vi "Obtain frame number and location-single bin file.vi"(8 "error in (no error)":errorcluster, 9 "Experiment Header's Statistics":T2, 10 "Acquisition time unknown":bool, 11 "Binary file to read":path) -> (0 "error out":errorcluster, 1 "Frame numbers & locations":T1)   [LabVIEW 2013]
uses:
  Typedefs/Test header stats cluster.ctl
  Typedefs/Number of frames and locations cluster.ctl
  Program Files (x86)/National Instruments/LabVIEW 2013/user.lib/_OpenG.lib/array/array.llb/Conditional Auto-Indexing Tunnel (I64)__ogtk.vi
panel:
  out "Frame size (bytes)":i64
  out "number of frames":dbl format="%#.6f"
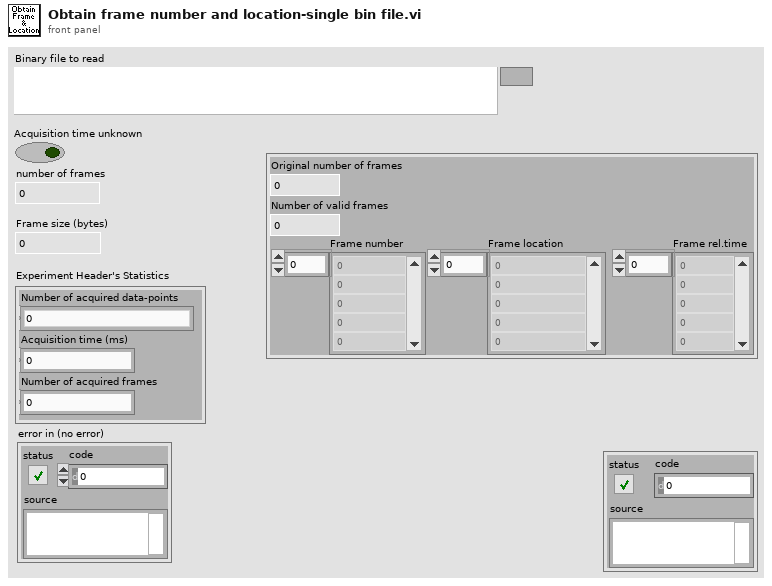
[diagram p1: front panel]
types:
  T1 = typedef "Number of frames and locations cluster.ctl" = cluster{"Original number of frames":i32, "Number of valid frames":i32, "Frame number":i64[], "Frame location":i64[], "Frame rel.time":i64[]}
  T2 = typedef "Test header stats cluster.ctl" = cluster{"Number of acquired data-points":dbl, "Acquisition time (ms)":dbl, "Number of acquired frames":dbl}
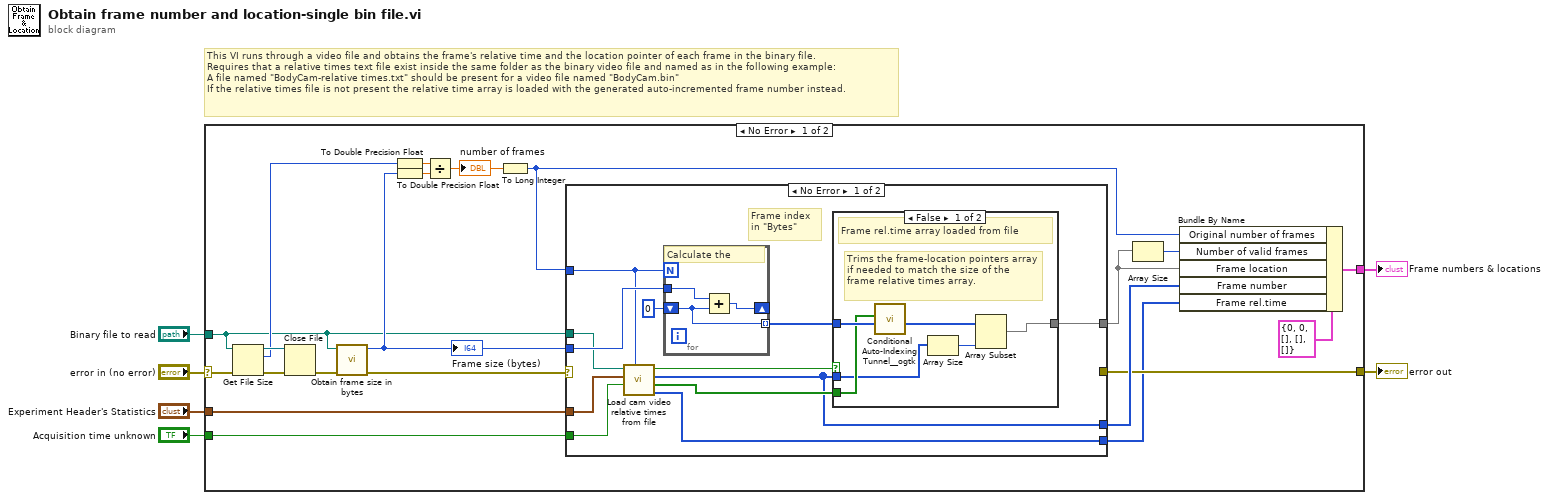
[diagram p0: block diagram]
diagram:
  # "This VI runs through a video file and obtains the frame's relative time and the location pointer of each frame in the binary file.\nRequires that a relative times text file exist inside the same folder as the binary video file and named as in the following example:\nA file named \"BodyCam-relative times.txt\" should be present for a video file named \"BodyCam.bin\"\nIf the relative times file is not present the relative time array is loaded with the generated auto-incremented frame number instead."
  n1 = case shown="No Error" "error in (no error)" {
    selector: "error in (no error)" -> [w16 w51]
    tunnel: "Binary file to read" -> [w14 _]
    tunnel: [w20 _] -> w1
    tunnel: [w19 w51] -> w4
    tunnel: "Experiment Header's Statistics" -> [w13 _]
    tunnel: "Acquisition time unknown" -> [w12 _]
    frame No Error {
      n2 = Get File Size(file=w14, error in=w16) -> (refnum out=w27:refnum<file>, size (in bytes)=w22:i64, 0:w26:errorcluster)
      n3 = Close File(refnum=w27, error in=w26) -> (error out=w18:errorcluster)  [unwired: 1 out]
      n4 = call "Obtain frame size in bytes.vi"("error in (no error)"=w18, "Binary file to read"=w14) -> ("error out"=w15:errorcluster, "Frame size (bytes)"=w17:i64)  [unwired: 8 in]
      "Frame size (bytes)" <- w17
      n5 = To Double Precision Float(number=w22) -> (double precision float=w23:dbl)
      n6 = To Double Precision Float(number=w17) -> (double precision float=w24:dbl)
      n7 = Divide(x=w23, y=w24) -> (x/y=w25:dbl)
      "number of frames" <- w25
      n8 = To Long Integer(number=w25) -> (32bit integer=w10:i32)
      n9 = case shown="No Error" w15 {
        selector: w15 -> [_ w50]
        tunnel: w10 -> [w31 _]
        tunnel: w17 -> [w39 _]
        tunnel: [w29 _] -> w21
        tunnel: [w36 _] -> w8
        tunnel: [_ w50] -> w19
        tunnel: w14 -> [w37 _]
        tunnel: w13 -> [w33 _]
        tunnel: w12 -> [w32 _]
        tunnel: [w28 _] -> w7
        frame No Error {
          # "Frame index in \"Bytes\""
          n10 = call "Load cam video relative times from file.vi"("Number of frames"=w31, "Acquisition time unknown"=w32, "Experiment Header's Statistics"=w33, "Binary file to read"=w37) -> ("Frame relative times array"=w28:i64[], "Elements to keep"=w30:bool[], "Frame numbers array"=w29:i64[], "Relative times file not found or error"=w34:bool)  [unwired: 4 in]
          n11 = for {
            N: w31 -> [_]
            tunnel: w39 -> [w48]
            shift-right: [w49] -> _
            shift-left: i64 0 -> [w47]
            tunnel: [w47] -> w35 mode=indexing
            # "Calculate the"
            n12 = Add(x=w48, y=w47) -> (x+y=w49:i64)
          }
          n13 = case shown="False" w34 {
            tunnel: [w44 w46] -> w36
            tunnel: w35 -> [w43 w46]
            tunnel: w30 -> [w41 _]
            tunnel: w29 -> [w40 _]
            frame False {
              # "Trims the frame-location pointers array if needed to match the size of the frame relative times array."
              # "Frame rel.time array loaded from file"
              n14 = call-poly "Conditional Auto-Indexing Tunnel__ogtk.vi"("Array in"=w43, "Elements to keep"=w41) -> ("Filtered Array out"=w42:i64[])  [unwired: 5 in]
              n15 = Array Size(array=w40) -> (size(s)=w45:i32)
              n16 = Array Subset(array=w42, length=w45) -> (w44:i64[])  [unwired: 1 in]
            }
            frame True {
              # "Frame rel.time array generated"
            }
          }
        }
        frame Error {
        }
      }
      n17 = Array Size(array=w8) -> (size(s)=w9:i32)
      n18 = Bundle By Name(cluster=T1 {"Original number of frames"=0, "Number of valid frames"=0, "Frame number"=[], "Frame location"=[], "Frame rel.time"=[]} ("Frame numbers & locations"), "Original number of frames"=w10, "Number of valid frames"=w9, "Frame location"=w8, "Frame number"=w21, "Frame rel.time"=w7) -> (w20:T1)
    }
    frame Error {
    }
  }
  "error out" <- w4
  "Frame numbers & locations" <- w1
